vi "resolve control references.vi"(4 "output dictionary":refnum<class "data dictionary.lvclass">, 6 "input dictionary":refnum<class "data dictionary.lvclass">, 8 "error in":errorcluster, 10 "UI Ref":refnum<vi>, 11 "channels in":refnum<class "TBM channel.lvclass">[](array[class])) -> (0 "error out":errorcluster, 2 "indicators":T1[](array[typedef]), 3 "controls":T1[](array[typedef]))   [LabVIEW 2015, in "UI Reference runtime.lvclass"]
uses:
  UI Reference runtime.lvclass
  <vilib>/NI/Tag Bus Module Framework/channel/TBM channel.lvclass
  control index set.ctl
  <vilib>/NI/Tag Bus/tag/Data Type.ctl
  <vilib>/NI/Tag Bus/dictionary/data dictionary.lvclass
  <vilib>/NI/Tag Bus Module Framework/channel/TBM channel.lvclass/TBM channel.ctl
  <vilib>/NI/Tag Bus/tag/tag descriptor.lvclass/tag descriptor.ctl
  <vilib>/NI/Tag Bus Module Framework/channel/Read channel classification.vi
  <vilib>/NI/Tag Bus/tag/read tag name.vi
  <vilib>/NI/Tag Bus/tag/read data type.vi
  <vilib>/NI/Tag Bus/tag/tag descriptor.lvclass
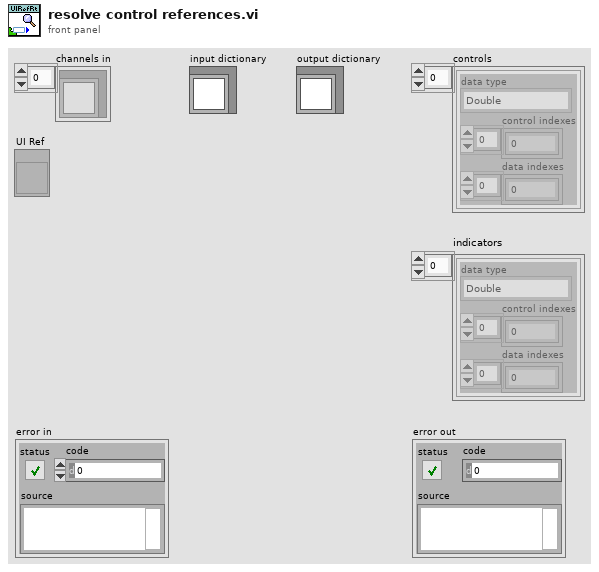
[diagram p1: front panel]
types:
  T1 = typedef "UI Reference runtime.lvclass/control index set.ctl" = cluster{"data type":T2, "control indexes":i32[], "data indexes":i32[]}
  T2 = typedef "tag bus.lvlib/tag descriptor.lvclass/Data Type.ctl" = enum16{"Double", "Single", "I64", "I32", "I16", "I8", "U64", "U32", "U16", "U8", "Boolean", "String", "Array of Double", "Array of Single", "Array of I64", "Array of I32", "Array of I16", "Array of I8", "Array of U64", "Array of U32", "Array of U16", "Array of U8", "Array of Boolean", "Array of String"}
  T3 = typedef "TBM channel.lvclass/channel classification.ctl" = enum16{"input data", "output data", "processing parameter", "processing result"}
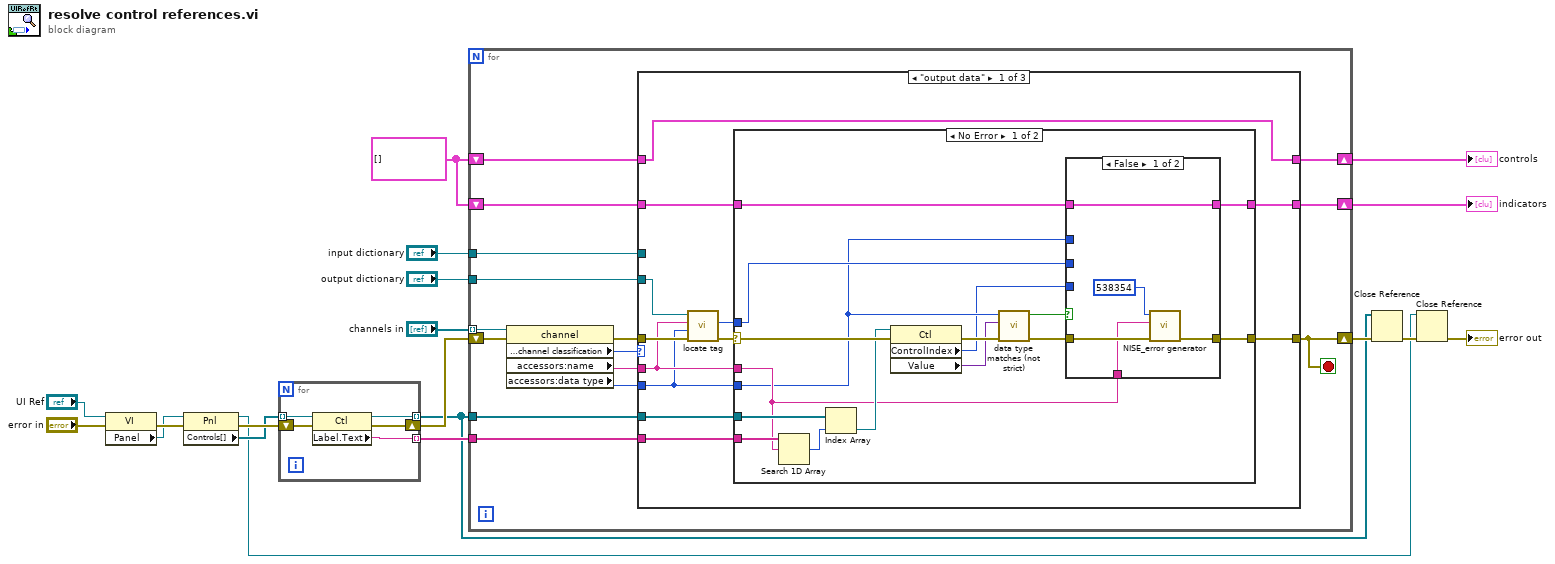
[diagram p0: block diagram]
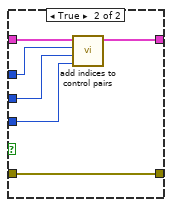
[diagram p2: hidden frame]
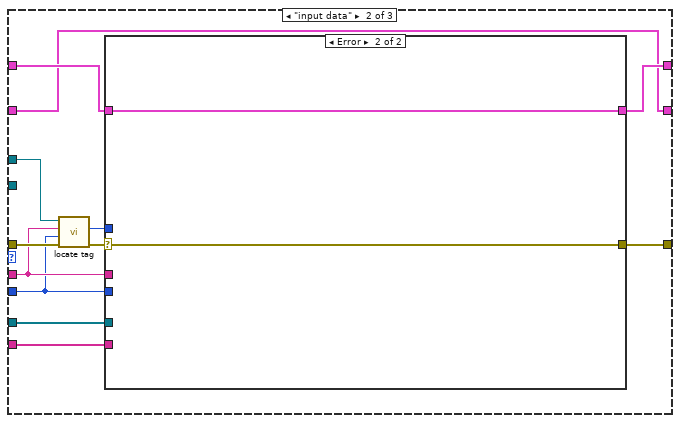
[diagram p4: hidden frame]
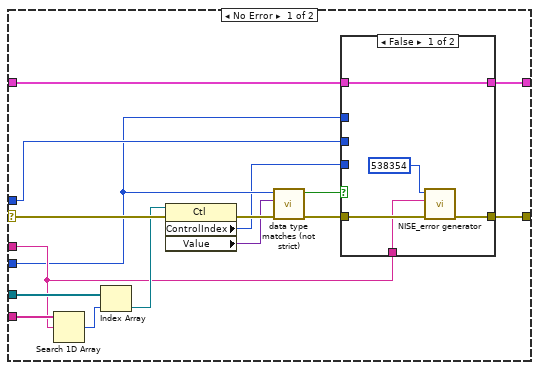
[diagram p5: hidden frame]
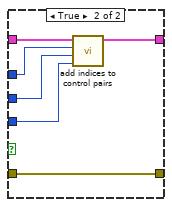
[diagram p6: hidden frame]
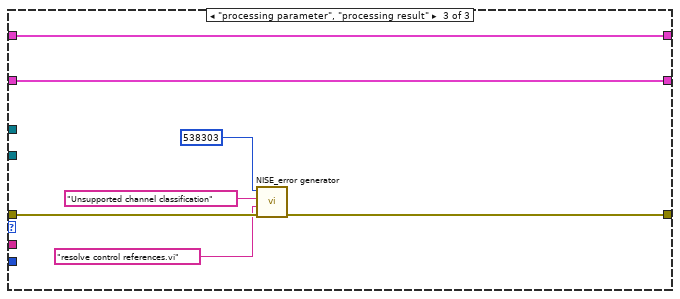
[diagram p7: hidden frame]
diagram:
  w10 = T1[] [] ("indicators")
  n1 = property class="VI"(reference="UI Ref", error in="error in") -> (error out=w16:errorcluster, "Panel"=w15:refnum<vi>)  [unwired: 1 out]
  n2 = property class="Pnl"(reference=w15, error in=w16) -> (reference out=w2:refnum<vi>, error out=w14:errorcluster, "Controls[]"=w13:refnum<vi>[])
  n3 = for {
    shift-right: [w22] -> w11
    shift-left: w14 -> [w23]
    tunnel: w13 -> [w24] mode=indexing
    tunnel: [w21] -> w12 mode=indexing
    tunnel: [w20] -> w1 mode=indexing
    n4 = property class="Ctl"(reference=w24, error in=w23) -> (reference out=w20:refnum<vi>, error out=w22:errorcluster, "Label.Text"=w21:string)
  }
  n5 = for {
    tunnel: "channels in" -> [w39] mode=indexing
    tunnel: w1 -> [w26]
    tunnel: w12 -> [w25]
    shift-right: [w34] -> w8
    shift-left: w10 -> [w33]
    shift-right: [w31] -> w7
    shift-left: w10 -> [w32]
    shift-right: [w35] -> w9
    shift-left: w11 -> [w38]
    tunnel: "output dictionary" -> [w27]
    tunnel: "input dictionary" -> [w30]
    stop <- w35 stop-if-true
    n6 = property class="channel"(reference=w39, error in=w38) -> (error out=w36:errorcluster, "data access:channel classification"=w37:T3, "accessors:name"=w29:string, "accessors:data type"=w28:T2)  [unwired: 1 out]
    n7 = case shown="\"output data\"" w37 {
      tunnel: w36 -> [w51 w92 w128]
      tunnel: [w46 w88 w126] -> w35
      tunnel: [w43 w82 w123] -> w34
      tunnel: w33 -> [w43 w83 w123]
      tunnel: w32 -> [w45 w81 w122]
      tunnel: [w44 w81 w122] -> w31
      tunnel: w30 -> [_ w84 _]
      tunnel: w29 -> [w48 w90 _]
      tunnel: w28 -> [w47 w89 _]
      tunnel: w27 -> [w50 _ _]
      tunnel: w26 -> [w41 w86 _]
      tunnel: w25 -> [w42 w87 _]
      frame "output data" {
        n8 = call <vilib>:"locate tag.vi"("error in"=w51, "data type"=w47, "name"=w48, "data dictionary in"=w50) -> ("error out"=w49:errorcluster, "index"=w40:i32)  [unwired: 5 in, 1 out]
        n9 = case shown="No Error" w49 {
          selector: w49 -> [w64 w80]
          tunnel: w48 -> [w57 _]
          tunnel: w47 -> [w53 _]
          tunnel: [w59 w80] -> w46
          tunnel: w45 -> [w55 w79]
          tunnel: [w56 w79] -> w44
          tunnel: w42 -> [w67 _]
          tunnel: w41 -> [w66 _]
          tunnel: w40 -> [w54 _]
          frame No Error {
            n10 = Search 1D Array(1D array=w67, element=w57) -> (index of element=w65:i32)  [unwired: 1 in]
            n11 = Index Array(array=w66, index=w65) -> (element=w63:refnum<vi>)
            n12 = property class="Ctl"(reference=w63, error in=w64) -> (error out=w62:errorcluster, "ControlIndex"=w52:i32, "Value"=w61:variant)  [unwired: 1 out]
            n13 = call "data type matches (not strict).vi"("error in"=w62, "Value"=w61, "data type"=w53) -> ("error out"=w58:errorcluster, "type match"=w60:bool)  [unwired: 7 in]
            n14 = case shown="False" w60 {
              tunnel: [w71 w78] -> w59
              tunnel: w58 -> [w70 w78]
              tunnel: w57 -> [w69 _]
              tunnel: [w68 w76] -> w56
              tunnel: w55 -> [w68 w77]
              tunnel: w54 -> [_ w74]
              tunnel: w53 -> [_ w75]
              tunnel: w52 -> [_ w73]
              frame False {
                n15 = call <vilib>:"NISE_error generator.vi"("error in"=w70, "append error message"=w69, "error code (0)"=538354) -> ("error out"=w71:errorcluster)  [unwired: 6 in]
              }
              frame True {
                n16 = call "add indices to control pairs.vi"("control index"=w73, "data index"=w74, "data type"=w75, "pairs in"=w77) -> ("pairs out"=w76:T1[])  [unwired: 7 in]
              }
            }
          }
          frame Error {
          }
        }
      }
      frame "input data" {
        n17 = call <vilib>:"locate tag.vi"("error in"=w92, "data type"=w89, "name"=w90, "data dictionary in"=w84) -> ("error out"=w91:errorcluster, "index"=w85:i32)  [unwired: 5 in, 1 out]
        n18 = case shown="Error" w91 {
          selector: w91 -> [w105 w121]
          tunnel: w90 -> [w98 _]
          tunnel: w89 -> [w94 _]
          tunnel: [w100 w121] -> w88
          tunnel: w83 -> [w96 w120]
          tunnel: [w97 w120] -> w82
          tunnel: w87 -> [w108 _]
          tunnel: w86 -> [w107 _]
          tunnel: w85 -> [w95 _]
          frame No Error {
            n19 = Search 1D Array(1D array=w108, element=w98) -> (index of element=w106:i32)  [unwired: 1 in]
            n20 = Index Array(array=w107, index=w106) -> (element=w104:refnum<vi>)
            n21 = property class="Ctl"(reference=w104, error in=w105) -> (error out=w103:errorcluster, "ControlIndex"=w93:i32, "Value"=w102:variant)  [unwired: 1 out]
            n22 = call "data type matches (not strict).vi"("error in"=w103, "Value"=w102, "data type"=w94) -> ("error out"=w99:errorcluster, "type match"=w101:bool)  [unwired: 7 in]
            n23 = case shown="False" w101 {
              tunnel: [w112 w119] -> w100
              tunnel: w99 -> [w111 w119]
              tunnel: w98 -> [w110 _]
              tunnel: [w109 w117] -> w97
              tunnel: w96 -> [w109 w118]
              tunnel: w95 -> [_ w115]
              tunnel: w94 -> [_ w116]
              tunnel: w93 -> [_ w114]
              frame False {
                n24 = call <vilib>:"NISE_error generator.vi"("error in"=w111, "append error message"=w110, "error code (0)"=538354) -> ("error out"=w112:errorcluster)  [unwired: 6 in]
              }
              frame True {
                n25 = call "add indices to control pairs.vi"("control index"=w114, "data index"=w115, "data type"=w116, "pairs in"=w118) -> ("pairs out"=w117:T1[])  [unwired: 7 in]
              }
            }
          }
          frame Error {
          }
        }
      }
      frame "processing parameter", "processing result" {
        n26 = call <vilib>:"NISE_error generator.vi"("error in"=w128, "source"="resolve control references.vi", "append error message"="Unsupported channel classification", "error code (0)"=538303) -> ("error out"=w126:errorcluster)  [unwired: 5 in]
      }
    }
  }
  "controls" <- w8
  "indicators" <- w7
  n27 = Close Reference(reference=w1, error in (no error)=w9) -> (error out=w4:errorcluster)
  n28 = Close Reference(reference=w2, error in (no error)=w4) -> (error out=→"error out":errorcluster)
